vi "QKD-BBM92.vi"() -> ()   [LabVIEW 2020]
uses:
  Gates/Polymorphs/vControl_e.vi
  Gates/Polymorphs/Pauli-X_t.vi
  Analysis/Inspect VIs/Entanglement Table - Display.vi
panel:
  out "Shots":i32=100
  out "QBER Meter":dbl(knob) scale=0.0..100.0
  out "Sifted Key Size":i32
  out "Bob's Sifted Key":bool[](array[boolean])
  out "Alice's Sifted Key":bool[](array[boolean])
  in  "Eavesdropper":bool
  # "BBM92 Protocol: Entanglement-Based QKD"
  # "This simulation demonstrates how quantum mechanics guarantees communication security.\n- Run the VI to generate a shared key.\n- Toggle the Eavesdropper to observe how the laws of physics prevent undetected interception."
  # "Eavesdropper (Eve) Interception\nOFF: The entangled state reaches Alice and Bob intact, ensuring perfect correlation when measured in the same basis.\nON: Eve intercepts the transmission! Her forced measurements prematurely collapse the shared wave function. The entanglement is severed, leaving behind only classical, uncorrelated photons."
  # "Quantum Bit Error Rate (QBER)\nMonitors the percentage of mismatched bits in the sifted keys.\n0%: Entanglement verified; the channel is secure.\n~25%: Entanglement broken! Eve's interception collapsed the quantum state, introducing a permanent, mathematically detectable error rate."
  # "The Sifted Keys (Correlated Results)\nAlice and Bob compare their publicly available random measurement bases and keep only the rounds where they matched. Because they measured an entangled state, their resulting bits are guaranteed to be identical, forming the shared secret key."
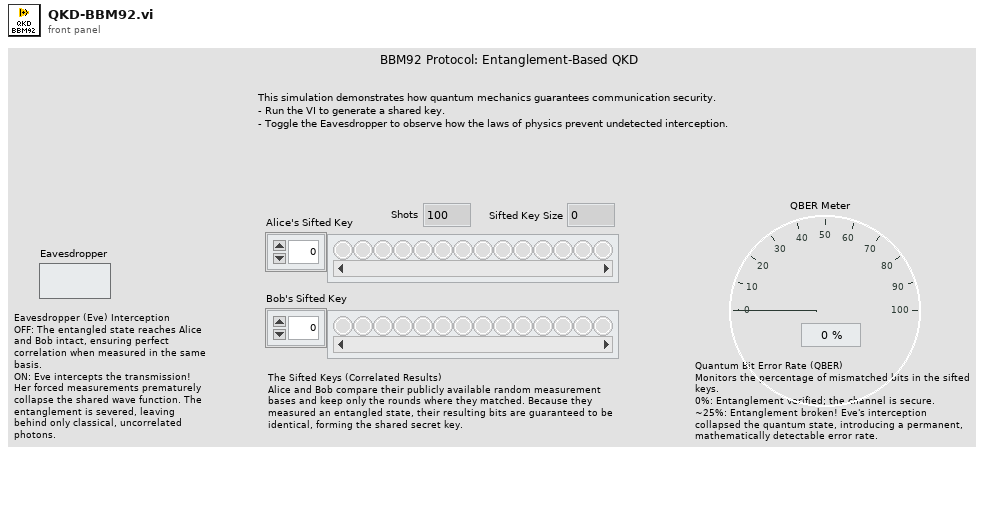
[diagram p1: front panel]
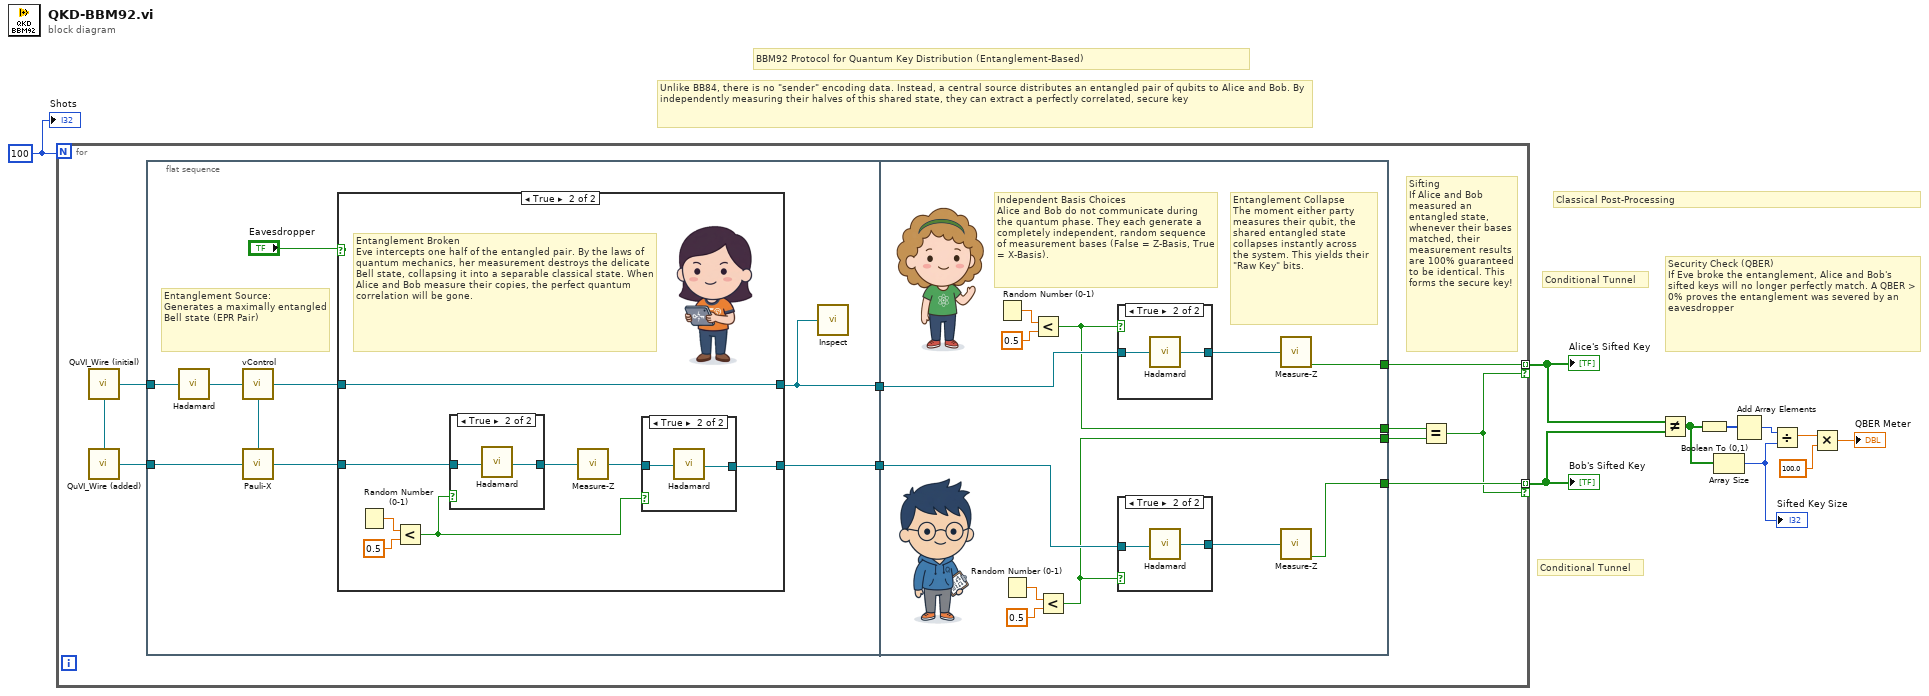
[diagram p0: block diagram]
diagram:
  w7 = 100
  # "Unlike BB84, there is no \"sender\" encoding data. Instead, a central source distributes an entangled pair of qubits to Alice and Bob. By independently measuring their halves of this shared state, they can extract a perfectly correlated, secure key"
  # "Conditional Tunnel"
  # "Conditional Tunnel"
  # "Security Check (QBER)\nIf Eve broke the entanglement, Alice and Bob's sifted keys will no longer perfectly match. A QBER > 0% proves the entanglement was severed by an eavesdropper"
  # "BBM92 Protocol for Quantum Key Distribution (Entanglement-Based)"
  # "Classical Post-Processing"
  n1 = for {
    N: w7 -> [_]
    tunnel: [w15] -> w3 mode=indexing if=w13
    tunnel: [w14] -> w4 mode=indexing if=w13
    # "Sifting\nIf Alice and Bob measured an entangled state, whenever their bases matched, their measurement results are 100% guaranteed to be identical. This forms the secure key!"
    n2 = call "QuVI_Wire (initial).vi"() -> ("QuWire out"=w19:refnum<class "QuWire.lvclass">, "Stack out"=w20:refnum<class "QuSim.lvclass">)  [unwired: 14 in]
    n3 = call "QuVI_Wire (added).vi"("Stack in"=w20) -> ("QuWire out"=w18:refnum<class "QuWire.lvclass">)  [unwired: 13 in, 1 out]
    n4 = flat-sequence {
      tunnel: w19 -> [w28]
      tunnel: w18 -> [w26]
      tunnel: [w23] -> w12
      tunnel: [w21] -> w11
      tunnel: [w49] -> w14
      tunnel: [w47] -> w15
      tunnel: [w46] -> w16
      tunnel: [w48] -> w17
      tunnel: w12 -> [w53]
      tunnel: w11 -> [w51]
      frame #0 {
        # "Entanglement Source:\nGenerates a maximally entangled Bell state (EPR Pair)"
        n5 = call "Hadamard.vi"("QuWire in"=w28) -> ("QuWire out"=w29:refnum<class "QuWire.lvclass">)  [unwired: 14 in]
        n6 = call-poly "vControl.vi"("QuWire in"=w29) -> ("QuWire out"=w22:refnum<class "QuWire.lvclass">, "v Ctrl out"=w27:refnum<class "CtrlLine.lvclass">)  [unwired: 13 in]
        n7 = call-poly "Pauli-X.vi"("v Ctrl  in"=w27, "QuWire in"=w26) -> ("QuWire out"=w24:refnum<class "QuWire.lvclass">)  [unwired: 13 in]
        n8 = case shown="True" "Eavesdropper" {
          tunnel: w24 -> [w31 w35]
          tunnel: [w31 w33] -> w23
          tunnel: w22 -> [w30 w36]
          tunnel: [w30 w36] -> w21
          frame False {
          }
          frame True {
            # "Entanglement Broken\nEve intercepts one half of the entangled pair. By the laws of quantum mechanics, her measurement destroys the delicate Bell state, collapsing it into a separable classical state. When Alice and Bob measure their copies, the perfect quantum correlation will be gone."
            n9 = Random Number (0-1)() -> (number: 0 to 1=w38:dbl)
            n10 = Less?(x=w38, y=0.5 ("x")) -> (x < y?=w32:bool)
            n11 = case shown="True" w32 {
              tunnel: w35 -> [w43 w45]
              tunnel: [w43 w44] -> w37
              frame False {
              }
              frame True {
                n12 = call "Hadamard.vi"("QuWire in"=w45) -> ("QuWire out"=w44:refnum<class "QuWire.lvclass">)  [unwired: 14 in]
              }
            }
            n13 = call "Measure-Z.vi"("QuWire in"=w37) -> ("QuWire out"=w34:refnum<class "QuWire.lvclass">)  [unwired: 13 in, 1 out]
            n14 = case shown="True" w32 {
              tunnel: w34 -> [w40 w42]
              tunnel: [w40 w41] -> w33
              frame False {
              }
              frame True {
                n15 = call "Hadamard.vi"("QuWire in"=w42) -> ("QuWire out"=w41:refnum<class "QuWire.lvclass">)  [unwired: 14 in]
              }
            }
          }
        }
        n16 = call-poly "Inspect.vi"("QuWire in"=w21) -> ()  [unwired: 15 in]
      }
      frame #1 {
        # "Entanglement Collapse\nThe moment either party measures their qubit, the shared entangled state collapses instantly across the system. This yields their \"Raw Key\" bits."
        # "Independent Basis Choices\nAlice and Bob do not communicate during the quantum phase. They each generate a completely independent, random sequence of measurement bases (False = Z-Basis, True = X-Basis)."
        n17 = Random Number (0-1)() -> (number: 0 to 1=w54:dbl)
        n18 = Random Number (0-1)() -> (number: 0 to 1=w56:dbl)
        n19 = Less?(x=w54, y=0.5 ("x")) -> (x < y?=w46:bool)
        n20 = Less?(x=w56, y=0.5 ("x")) -> (x < y?=w48:bool)
        n21 = case shown="True" w46 {
          tunnel: w51 -> [w61 w63]
          tunnel: [w61 w62] -> w55
          frame False {
          }
          frame True {
            n22 = call "Hadamard.vi"("QuWire in"=w63) -> ("QuWire out"=w62:refnum<class "QuWire.lvclass">)  [unwired: 14 in]
          }
        }
        n23 = case shown="True" w48 {
          tunnel: w53 -> [w58 w60]
          tunnel: [w58 w59] -> w57
          frame False {
          }
          frame True {
            n24 = call "Hadamard.vi"("QuWire in"=w60) -> ("QuWire out"=w59:refnum<class "QuWire.lvclass">)  [unwired: 14 in]
          }
        }
        n25 = call "Measure-Z.vi"("QuWire in"=w55) -> ("Classical bit"=w47:bool)  [unwired: 13 in, 1 out]
        n26 = call "Measure-Z.vi"("QuWire in"=w57) -> ("Classical bit"=w49:bool)  [unwired: 13 in, 1 out]
      }
    }
    n27 = Equal?(x=w16, y=w17) -> (x = y?=w13:bool)
  }
  "Alice's Sifted Key" <- w3
  "Bob's Sifted Key" <- w4
  n28 = Not Equal?(x=w3, y=w4) -> (x != y?=w5:bool[])
  n29 = Boolean To (0,1)(Boolean=w5) -> (0, 1=w6:i16[])
  n30 = Array Size(array=w5) -> (size(s)=w2:i32)
  "Sifted Key Size" <- w2
  n31 = Add Array Elements(numeric array=w6) -> (sum=w10:i16)
  n32 = Divide(x=w10, y=w2) -> (x/y=w9:dbl)
  n33 = Multiply(x=w9, y=100.0) -> (x*y=→"QBER Meter":dbl)
  "Shots" <- w7
